vi "get_data_by_time.vi"(1 "Sample Rate":dbl=1000.0, 2 "横轴（显示时长）":dbl=1000.0, 3 "appended array":dbl[][][](array[numeric])) -> (6 "data":waveform(dbl)[](array[waveform]), 9 "new array":dbl[][][](array[numeric]))   [LabVIEW 2024]
panel:
  in  "Number of Samples":i32=100
  out "max page number":dbl
  out "sample number":i32
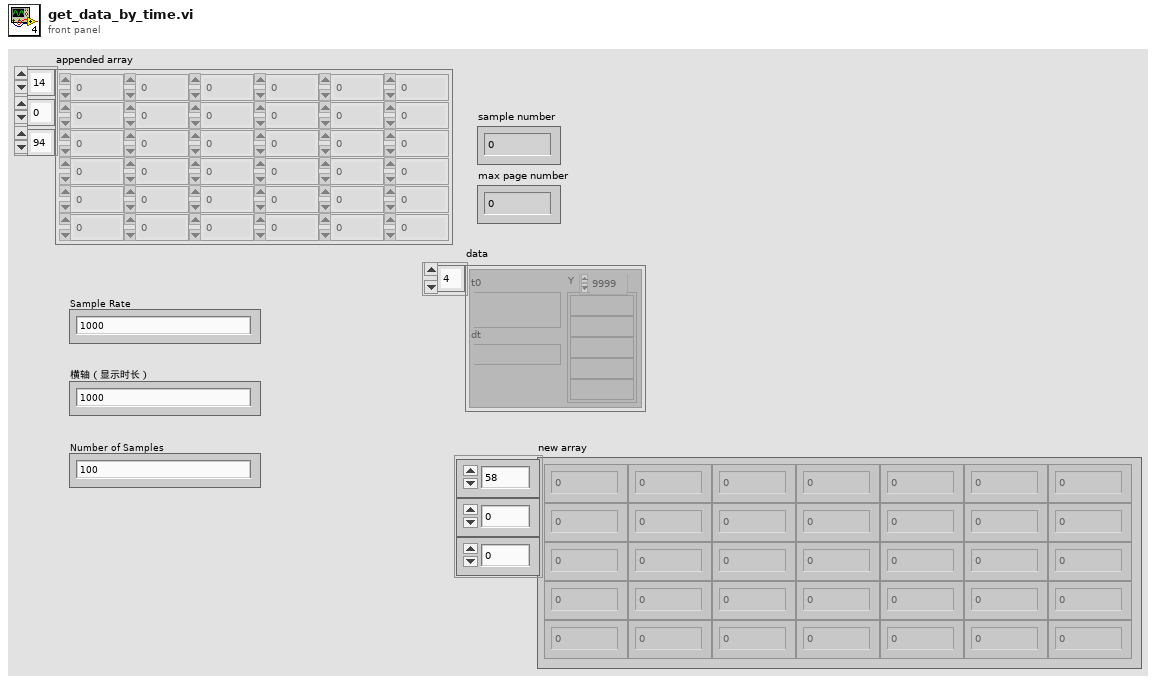
[diagram p1: front panel]
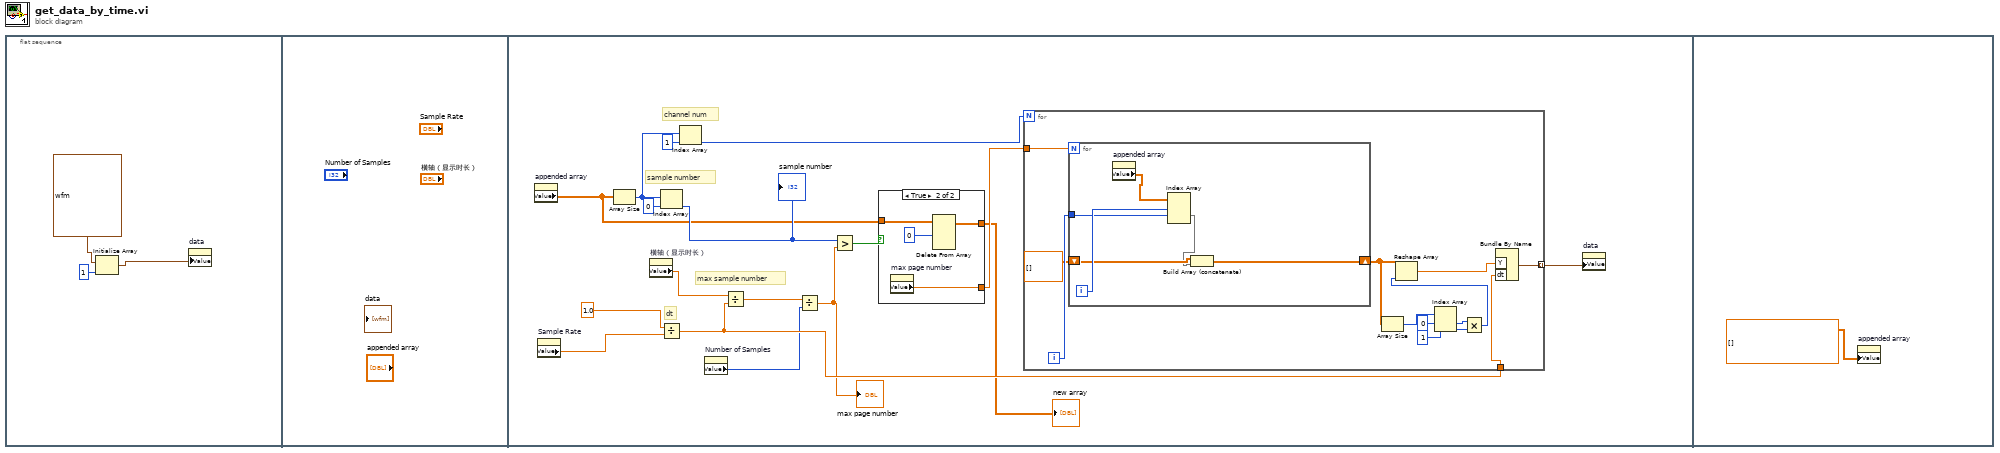
[diagram p0: block diagram]
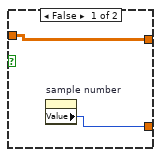
[diagram p2: hidden frame]
diagram:
  n1 = flat-sequence {
    frame #0 {
      n2 = Initialize Array(waveform(dbl) {"t0"=timestamp(0 s since 1904-01-01), "dt"=0.001, "Y"=array[245900 elements]} ("Waveform"), 1 ("dimension size")) -> (w3:waveform(dbl)[])
      n3 = property on="data" class="Arr (strict)"("Value"=w3) -> ()  [unwired: 2 in, 2 out]
    }
    frame #1 {
    }
    frame #2 {
      # "channel num"
      # "sample number"
      # "max sample number"
      # "dt"
      n4 = property on="appended array" class="Arr (strict)"() -> ("Value"=w8:dbl[][][])  [unwired: 2 in, 2 out]
      n5 = property on="Sample Rate" class="DigNum (strict)"() -> ("Value"=w19:dbl)  [unwired: 2 in, 2 out]
      n6 = Array Size(array=w8) -> (size(s)=w14:i32[])
      n7 = property on="横轴（显示时长）" class="DigNum (strict)"() -> ("Value"=w18:dbl)  [unwired: 2 in, 2 out]
      n8 = Index Array(array=w14, index=0) -> (element=w16:i32)
      "sample number" <- w16
      n9 = Divide(x=1.0, y=w19) -> (x/y=w10:dbl)
      n10 = Index Array(array=w14, index=1) -> (element=w12:i32)
      n11 = property on="Number of Samples" class="DigNum (strict)"() -> ("Value"=w6:i32)  [unwired: 2 in, 2 out]
      n12 = Divide(x=w18, y=w10) -> (x/y=w5:dbl)
      n13 = Divide(x=w5, y=w6) -> (x/y=w4:dbl)
      "max page number" <- w4
      n14 = Greater?(x=w16, y=w4) -> (0:w15:bool)
      n15 = case shown="True" w15 {
        tunnel: w8 -> [w41 w45]
        tunnel: [w41 w43] -> w7
        tunnel: [w40 w42] -> w11
        frame False {
          n16 = property on="sample number" class="DigNum (strict)"() -> ("Value"=w40:i32)  [unwired: 2 in, 2 out]
        }
        frame True {
          n17 = property on="max page number" class="DigNum (strict)"() -> ("Value"=w42:dbl)  [unwired: 2 in, 2 out]
          n18 = Delete From Array(array=w45, index (dim 0)=0 ("index (page)")) -> (array with subset deleted=w43:dbl[][][])  [unwired: 3 in, 1 out]
        }
      }
      "new array" <- w7
      n19 = for {
        N: w12 -> [_]
        tunnel: w11 -> [w33]
        tunnel: w10 -> [w32]
        tunnel: [w31] -> w9 mode=indexing
        i -> [w30]
        n20 = for {
          N: w33 -> [_]
          tunnel: w30 -> [w37]
          shift-right: [w36] -> w28
          shift-left: dbl[][] [] -> [w35]
          i -> [w38]
          n21 = property on="appended array" class="Arr (strict)"() -> ("Value"=w39:dbl[][][])  [unwired: 2 in, 2 out]
          n22 = Index Array(array=w39, index (dim 0)=w38, index (dim 1)=w37) -> (element=w34:dbl[])  [unwired: 1 in]
          n23 = Build Array (concatenate)(w35, w34) -> (w36:dbl[][])
        }
        n24 = Array Size(array=w28) -> (size(s)=w27:i32[])
        n25 = Index Array(array=w27, index #1=0 ("index"), index #2=1 ("index")) -> (element #1=w26:i32, element #2=w21:i32)
        n26 = Multiply(x=w26, y=w21) -> (x*y=w25:i32)
        n27 = Reshape Array(w28, w25) -> (w29:dbl[])
        n28 = Bundle By Name("Y"=w29, "dt"=w32) -> (w31:waveform(dbl))  [unwired: 1 in]
      }
      n29 = property on="data" class="Arr (strict)"("Value"=w9) -> ()  [unwired: 2 in, 2 out]
    }
    frame #3 {
      n30 = property on="appended array" class="Arr (strict)"("Value"=dbl[][][] [] ("appended array")) -> ()  [unwired: 2 in, 2 out]
    }
  }
